vi "Get Number of Queued Commands.vi"(8 "error in (no error)":errorcluster, 11 "Command Processor Actor in":refnum<class "Command Processor Actor.lvclass">) -> (0 "error out":errorcluster, 2 "Number Queued Commands":i32, 3 "Command Processor Actor out":refnum<class "Command Processor Actor.lvclass">)   [LabVIEW 2014, in "Robot Actor Framework.lvlib" / "Command Processor Actor.lvlib" / "Command Processor Actor.lvclass"]
uses:
  Command Processor Actor.lvclass
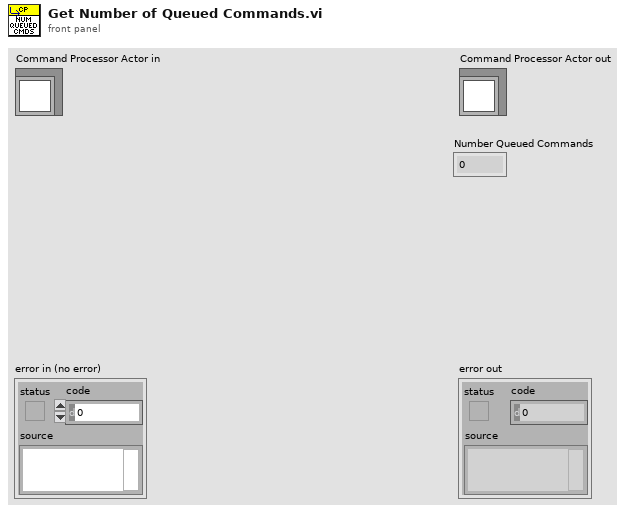
[diagram p1: front panel]
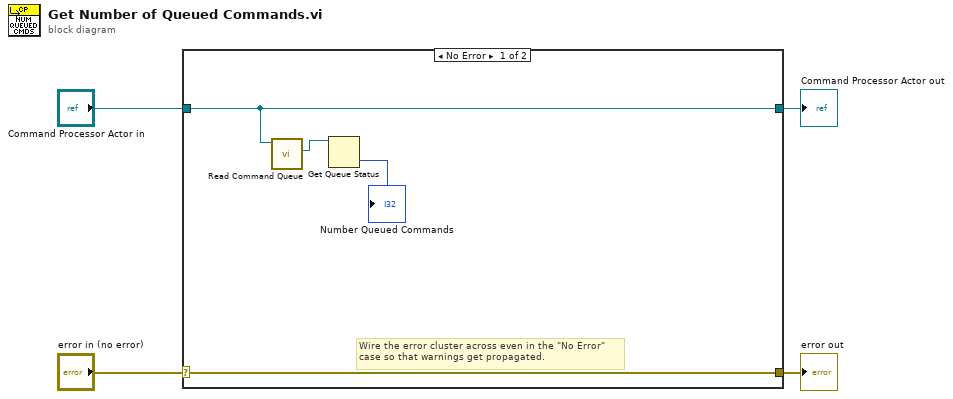
[diagram p0: block diagram]
diagram:
  n1 = case shown="No Error" "error in (no error)" {
    selector: "error in (no error)" -> [w8 w10]
    tunnel: [w8 w10] -> w3
    tunnel: [w7 w9] -> w1
    tunnel: "Command Processor Actor in" -> [w7 w9]
    frame No Error {
      # "Wire the error cluster across even in the \"No Error\"\ncase so that warnings get propagated."
      n2 = call-dynamic "Read Command Queue.vi"("Command Processor Actor in"=w7) -> ("Queued Commands"=w6:refnum<queue>)  [unwired: 8 in, 2 out]
      n3 = Get Queue Status(queue=w6) -> (# elements in queue=→"Number Queued Commands":i32)  [unwired: 2 in, 7 out]
    }
    frame Error {
    }
  }
  "error out" <- w3
  "Command Processor Actor out" <- w1
